vi "Get Update List.vi"(8 "error in (no error)":errorcluster, 10 "Filter FK/PK":T3, 11 "Update Fields Logic Simple Table in":refnum<class "Update Fields Logic Simple Table.lvclass">) -> (0 "error out":errorcluster, 2 "Fields to update":T1, 3 "Update Fields Logic Simple Table out":refnum<class "Update Fields Logic Simple Table.lvclass">)   [LabVIEW 2020, in "Update Fields Logic Simple Table.lvlib" / "Update Fields Logic Simple Table.lvclass"]
uses:
  Update Fields Logic Simple Table.lvclass
  Field FK PK Info.ctl
  Form FK Fields.ctl
  Form ID.ctl
  Update Fields Logic Simple Table.lvclass/Update Fields Logic Simple Table.ctl
  <userlib>/_OpenG.lib/array/array.llb/Search 1D Array (String)__ogtk.vi
  <userlib>/_OpenG.lib/array/array.llb/Index 1D Array Elements (String)__ogtk.vi
  <userlib>/_OpenG.lib/array/array.llb/Index 1D Array Elements (Variant)__ogtk.vi
  Form Server Interfaces.lvlib
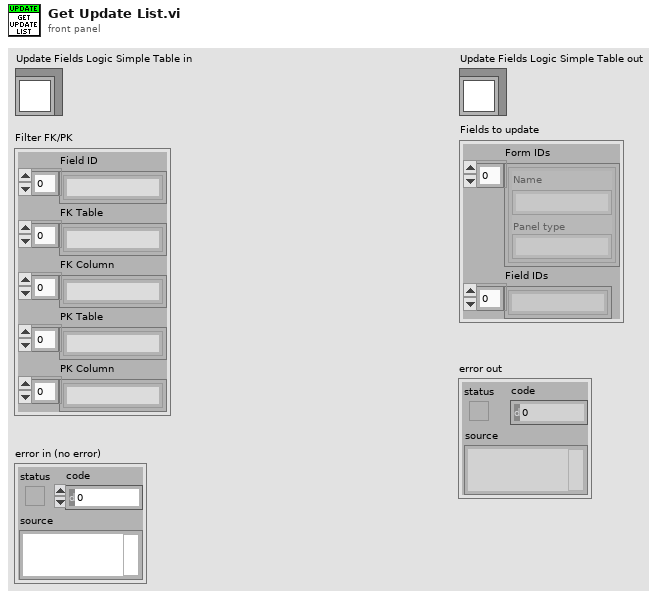
[diagram p1: front panel]
types:
  T1 = typedef "Form Server Interfaces.lvlib/Form FK Fields.ctl" = cluster{"Form IDs":T2[], "Field IDs":string[]}
  T2 = typedef "Form Server Interfaces.lvlib/Form ID.ctl" = cluster{"Name":string, "Panel type":string}
  T3 = typedef "Form Server Interfaces.lvlib/Field FK PK Info.ctl" = cluster{"Field ID":string[], "FK Table":string[], "FK Column":string[], "PK Table":string[], "PK Column":string[]}
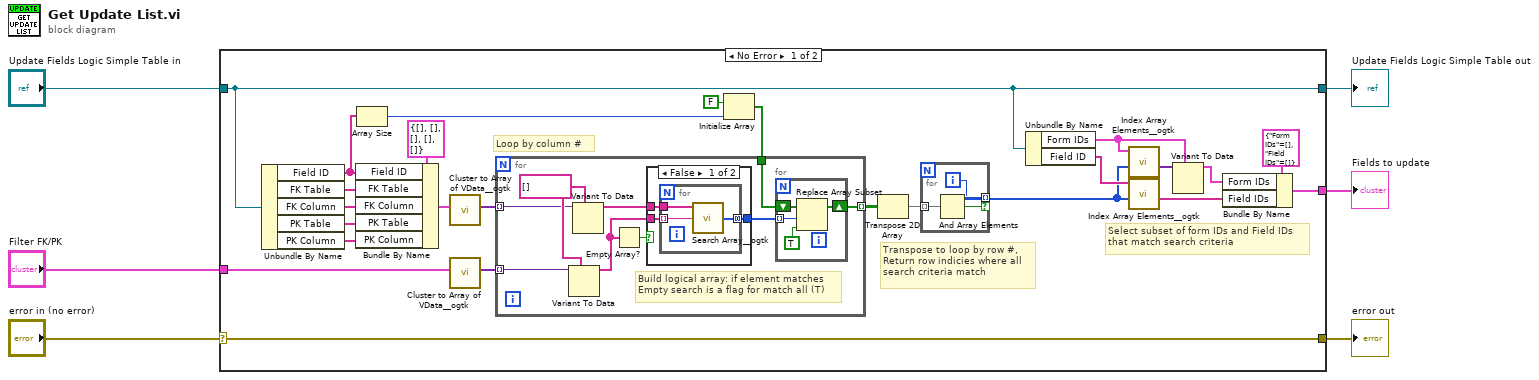
[diagram p0: block diagram]
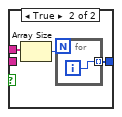
[diagram p2: hidden frame]
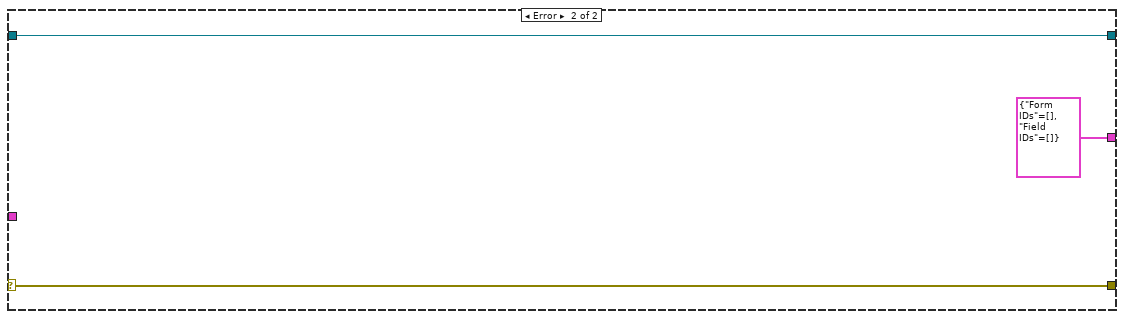
[diagram p3: hidden frame]
diagram:
  n1 = case shown="No Error" "error in (no error)" {
    selector: "error in (no error)" -> [w11 w60]
    tunnel: [w11 w60] -> w5
    tunnel: "Update Fields Logic Simple Table in" -> [w16 w59]
    tunnel: [w16 w59] -> w3
    tunnel: "Filter FK/PK" -> [w25 _]
    tunnel: [w7 T1 {"Form IDs"=[], "Field IDs"=[]} ("Fields to update")] -> w1
    frame No Error {
      # "Select subset of form IDs and Field IDs\nthat match search criteria"
      # "Loop by column #"
      # "Transpose to loop by row #,\nReturn row indicies where all\nsearch criteria match"
      n2 = Unbundle By Name(w16) -> ("Field ID"=w21:string[], "FK Table"=w30:string[], "FK Column"=w29:string[], "PK Table"=w28:string[], "PK Column"=w27:string[])
      n3 = Bundle By Name(cluster=T3 {"Field ID"=[], "FK Table"=[], "FK Column"=[], "PK Table"=[], "PK Column"=[]} ("FK/PK Info"), "Field ID"=w21, "FK Table"=w30, "FK Column"=w29, "PK Table"=w28, "PK Column"=w27) -> (w26:T3)
      n4 = Array Size(array=w21) -> (size(s)=w20:i32)
      n5 = call <userlib>:"Cluster to Array of VData__ogtk.vi"("Cluster"=w26) -> ("Array of VData"=w22:variant[])  [unwired: 9 in, 1 out]
      n6 = call <userlib>:"Cluster to Array of VData__ogtk.vi"("Cluster"=w25) -> ("Array of VData"=w24:variant[])  [unwired: 9 in, 1 out]
      n7 = Initialize Array(FALSE, w20) -> (w19:bool[])
      n8 = for {
        tunnel: w22 -> [w41] mode=indexing
        tunnel: w24 -> [w40] mode=indexing
        tunnel: w19 -> [w39]
        tunnel: [w38] -> w18 mode=indexing
        w43 = string[] []
        # "Build logical array: if element matches\nEmpty search is a flag for match all (T)"
        n9 = Variant To Data(type=w43, Variant=w40) -> (data=w36:string[])  [unwired: 1 in, 1 out]
        n10 = Variant To Data(type=w43, Variant=w41) -> (data=w42:string[])  [unwired: 1 in, 1 out]
        n11 = Empty Array?(array=w36) -> (empty?=w35:bool)
        n12 = case shown="False" w35 {
          tunnel: w42 -> [w46 w52]
          tunnel: [w45 w50] -> w37
          tunnel: w36 -> [w44 _]
          frame False {
            n13 = for {
              tunnel: w46 -> [w49]
              tunnel: [w48] -> w45 mode=concatenating
              tunnel: w44 -> [w47] mode=indexing
              n14 = call-poly <userlib>:"Search Array__ogtk.vi"("Array"=w49, "Element Data"=w47) -> ("Indices of Elements"=w48:i32[])  [unwired: 7 in]
            }
          }
          frame True {
            n15 = Array Size(array=w52) -> (size(s)=w51:i32)
            n16 = for {
              N: w51 -> [_]
              tunnel: [w53] -> w50 mode=indexing
              i -> [w53]
            }
          }
        }
        n17 = for {
          tunnel: w37 -> [w57] mode=indexing
          shift-right: [w54] -> w38
          shift-left: w39 -> [w56]
          n18 = Replace Array Subset(array=w56, new element=TRUE, index=w57) -> (w54:bool[])
        }
      }
      n19 = Transpose 2D Array(2D array=w18) -> (transposed array=w17:bool[][])
      n20 = for {
        tunnel: w17 -> [w34] mode=indexing
        tunnel: [w33] -> w14 mode=indexing if=w32
        i -> [w33]
        n21 = And Array Elements(Boolean array=w34) -> (logical AND=w32:bool)
      }
      n22 = Unbundle By Name(w16) -> ("Form IDs"=w12:T2[], "Field ID"=w15:string[])
      n23 = call-poly <userlib>:"Index Array Elements__ogtk.vi"("indices"=w14, "array"=w12) -> ("elements"=w13:variant[])  [unwired: 9 in]
      n24 = call-poly <userlib>:"Index Array Elements__ogtk.vi"("indices"=w14, "array"=w15) -> ("elements"=w8:string[])  [unwired: 9 in]
      n25 = Variant To Data(type=w12, Variant=w13) -> (data=w9:T2[])  [unwired: 1 in, 1 out]
      n26 = Bundle By Name(cluster=T1 {"Form IDs"=[], "Field IDs"=[]} ("Fields to update"), "Form IDs"=w9, "Field IDs"=w8) -> (w7:T1)
    }
    frame Error {
    }
  }
  "error out" <- w5
  "Update Fields Logic Simple Table out" <- w3
  "Fields to update" <- w1
